vi "Data retrieve engine_SE.vi"(0 "File or Folder Path":path=path "C:/Users/voodoo/Desktop/IV_separat_Vsgsweep_2fields_Vbg-2.8V", 5 "Scan names":string[](array[string]), 7 "IV setup":T2={"# of Vslow"=1, "# Vfast"=1, "#IV Curves at each gate"=2, "B/T offset"=0, "Discard first # curves"=1, "Manual offset"=0}, 9 "index":T3={"A"=3, "B"=4, "C"=2, "D"=4, "E"=3, "N1"=2, "N2"=2, "N3"=3, "N4"=4, "A 1"=8, "A 2"=14, "C 1"=5, "C 2"=1, "E 2"=4}, 11 "Portion of data":cluster{dbl, dbl}(slide)={0.75, 0.25} scale=0.0..1.0, 12 "Decimate point":dbl=1e-10 format="%#_1f", 13 "Extract paramaters from comments?":bool) -> (3 "Comments":string, 4 "IV":cluster{dbl[], dbl[]}[][](array[cluster])=[[{[-2.301174301585294e-09, -2.201174301585294e-09, -2.1011743015852944e-09, -2.0011743015852943e-09, -1.9011743015852942e-09, -1.8011743015852941e-09, -1.701174301585294e-09, -1.601174301585294e-09, -1.5011743015852941e-09, -1.401174301585294e-09, -1.301174301585294e-09, -1.2011743015852942e-09, -1.101174301585294e-09, -1.001174301585294e-09, -9.011743015852942e-10, -8.011743015852941e-10, -7.01174301585294e-10, -6.011743015852942e-10, -5.011743015852941e-10, -4.01174301585294e-10, -3.0117430158529395e-10, -2.0117430158529388e-10, -1.0117430158529423e-10, -1.1743015852941594e-12], [-2.4075285232756958e-05, -1.737972813858452e-05, -1.1037615852397166e-05, -5.267782040080203e-06, 2.4232289247411676e-07, 5.628820057942294e-06, 1.015781505747205e-05, 1.4463328409568988e-05, 1.817222828467457e-05, 2.105509970958606e-05, 2.409775741426245e-05, 2.720796229813868e-05, 3.0197002730537915e-05, 3.3043546244784785e-05, 3.5385544630750595e-05, 3.756777735485851e-05, 3.987253185589809e-05, 4.20620889081888e-05, 4.4006459573108544e-05, 4.587698979226302e-05, 4.7931581768717136e-05, 4.925252522526536e-05, 5.0480327825776546e-05, 8.08077413503745e-08]}]], 6 "IV-2T":cluster{dbl[], dbl[]}[][](array[cluster])=[[{[-2.301174301585294e-09, -2.201174301585294e-09, -2.1011743015852944e-09, -2.0011743015852943e-09, -1.9011743015852942e-09, -1.8011743015852941e-09, -1.701174301585294e-09, -1.601174301585294e-09, -1.5011743015852941e-09, -1.401174301585294e-09, -1.301174301585294e-09, -1.2011743015852942e-09, -1.101174301585294e-09, -1.001174301585294e-09, -9.011743015852942e-10, -8.011743015852941e-10, -7.01174301585294e-10, -6.011743015852942e-10, -5.011743015852941e-10, -4.01174301585294e-10, -3.0117430158529395e-10, -2.0117430158529388e-10, -1.0117430158529423e-10, -1.1743015852941594e-12], [-0.002353462043255516, -0.002297777119659299, -0.002239582947886705, -0.0021846959913649658, -0.0021298090348432263, -0.0020715829478867047, -0.0020166959913649656, -0.0019611544893886803, -0.0019081505368195105, -0.0018609817056506796, -0.0018106102770792509, -0.0017577829478867043, -0.001702609034843226, -0.001644382947886704, -0.001589759034843226, -0.001532834880253854, -0.001467967102476076, -0.0013968026580316317, -0.0013115945420896027, -0.0012138299473531684, -0.00047154515277183454, 0.001680737250983384, 0.0029627659595722446, 4.901687369444213e-06]}]], 8 "Vfast":dbl[][](array[numeric])=[[-1.3]], 10 "Vslow":dbl[](array[numeric])=[-1.3], 14 "N":cluster{"N1":dbl, "N2":dbl, "N3":dbl, "N4":dbl}={"N1"=8999.947, "N2"=0.049942, "N3"=-1.324126602495439e-06, "N4"=0.08912017346699704}, 15 "Vslowest":dbl)   [LabVIEW 2016]
uses:
  <vilib>/addons/WireFlow/_WF_ProgressBar.llb/ProgressBar_WireFlow.lvclass
  <vilib>/Analysis/2dsp.llb/Decimate (single shot, DBL).vi
  <vilib>/Analysis/NI_AALPro.lvlib
panel:
  in  "output array":path[](array[path])
  out "WF-ProgressBar out":refnum<class "ProgressBar_WireFlow.lvclass">
  in  "Tab Control":T1(tab)
  out "IV 2T":cluster{dbl[], dbl[]}[](graph)=[{[-2.301174301585294e-09, -2.201174301585294e-09, -2.1011743015852944e-09, -2.0011743015852943e-09, -1.9011743015852942e-09, -1.8011743015852941e-09, -1.701174301585294e-09, -1.601174301585294e-09, -1.5011743015852941e-09, -1.401174301585294e-09, -1.301174301585294e-09, -1.2011743015852942e-09, -1.101174301585294e-09, -1.001174301585294e-09, -9.011743015852942e-10, -8.011743015852941e-10, -7.01174301585294e-10, -6.011743015852942e-10, -5.011743015852941e-10, -4.01174301585294e-10, -3.0117430158529395e-10, -2.0117430158529388e-10, -1.0117430158529423e-10, -1.1743015852941594e-12], [-0.002353462043255516, -0.002297777119659299, -0.002239582947886705, -0.0021846959913649658, -0.0021298090348432263, -0.0020715829478867047, -0.0020166959913649656, -0.0019611544893886803, -0.0019081505368195105, -0.0018609817056506796, -0.0018106102770792509, -0.0017577829478867043, -0.001702609034843226, -0.001644382947886704, -0.001589759034843226, -0.001532834880253854, -0.001467967102476076, -0.0013968026580316317, -0.0013115945420896027, -0.0012138299473531684, -0.00047154515277183454, 0.001680737250983384, 0.0029627659595722446, 4.901687369444213e-06]}]
  out "IV":cluster{dbl[], dbl[]}[](graph)=[{[-2.301174301585294e-09, -2.201174301585294e-09, -2.1011743015852944e-09, -2.0011743015852943e-09, -1.9011743015852942e-09, -1.8011743015852941e-09, -1.701174301585294e-09, -1.601174301585294e-09, -1.5011743015852941e-09, -1.401174301585294e-09, -1.301174301585294e-09, -1.2011743015852942e-09, -1.101174301585294e-09, -1.001174301585294e-09, -9.011743015852942e-10, -8.011743015852941e-10, -7.01174301585294e-10, -6.011743015852942e-10, -5.011743015852941e-10, -4.01174301585294e-10, -3.0117430158529395e-10, -2.0117430158529388e-10, -1.0117430158529423e-10, -1.1743015852941594e-12], [-2.4075285232756958e-05, -1.737972813858452e-05, -1.1037615852397166e-05, -5.267782040080203e-06, 2.4232289247411676e-07, 5.628820057942294e-06, 1.015781505747205e-05, 1.4463328409568988e-05, 1.817222828467457e-05, 2.105509970958606e-05, 2.409775741426245e-05, 2.720796229813868e-05, 3.0197002730537915e-05, 3.3043546244784785e-05, 3.5385544630750595e-05, 3.756777735485851e-05, 3.987253185589809e-05, 4.20620889081888e-05, 4.4006459573108544e-05, 4.587698979226302e-05, 4.7931581768717136e-05, 4.925252522526536e-05, 5.0480327825776546e-05, 8.08077413503745e-08]}]
  # "Use to extract gate values in comments\neg. Vsg1="
  # "Default:\n4 terminal V vs I \n2 terminal V vs I"
  # "How many curves at each field/temperature? Usually should be N(Vslow)*N(Vfast)*N(each gate)"
  # "Discard first few IV curves at each gate if the gate need\ntime to settle"
  # "Default decimate on current axis instead of voltage axis. Decimation is needed for extracting dV/dI"
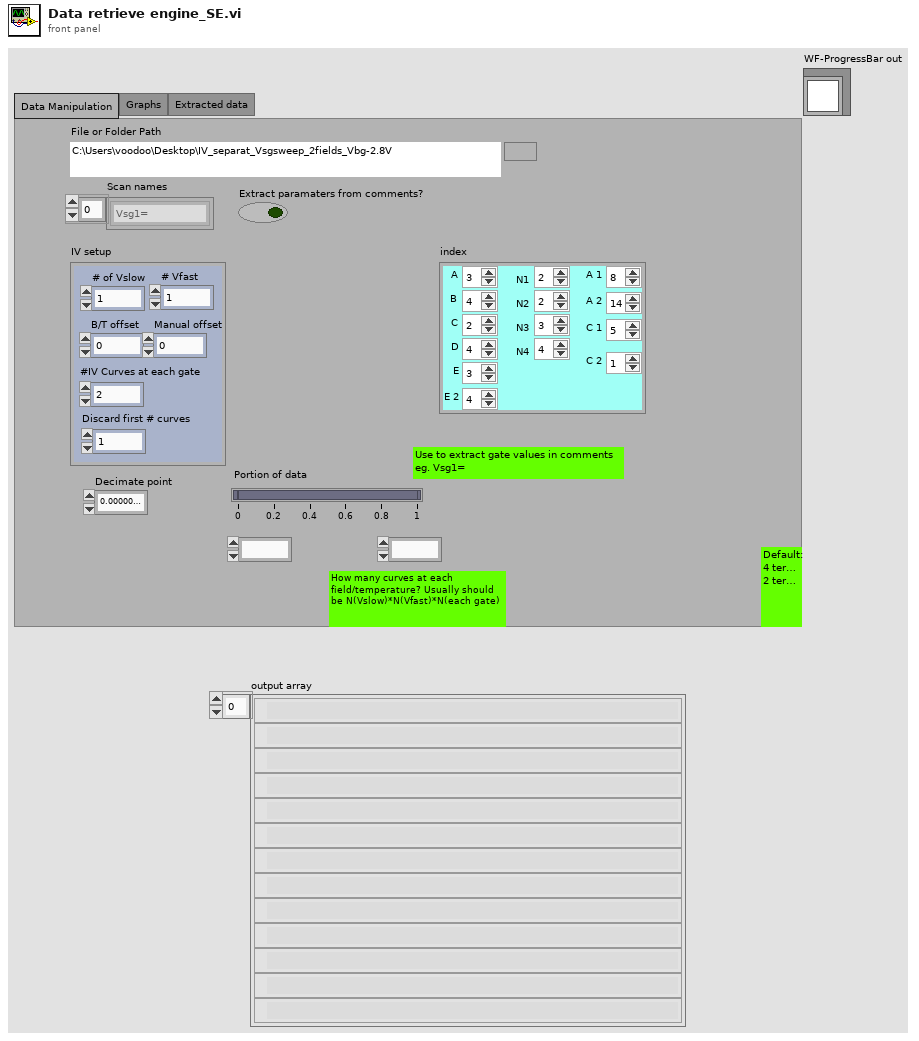
[diagram p1: front panel]
types:
  T1 = enum32{"Data Manipulation", "Graphs", "Extracted data"}
  T2 = cluster{"# of Vslow":i32, "# Vfast":i32, "#IV Curves at each gate":i32, "B/T offset":i32, "Discard first # curves":i32, "Manual offset":i32}
  T3 = cluster{"A":i32, "B":i32, "C":i32, "D":i32, "E":i32, "N1":i32, "N2":i32, "N3":i32, "N4":i32, "A 1":i32, "A 2":i32, "C 1":i32, "C 2":i32, "E 2":i32}
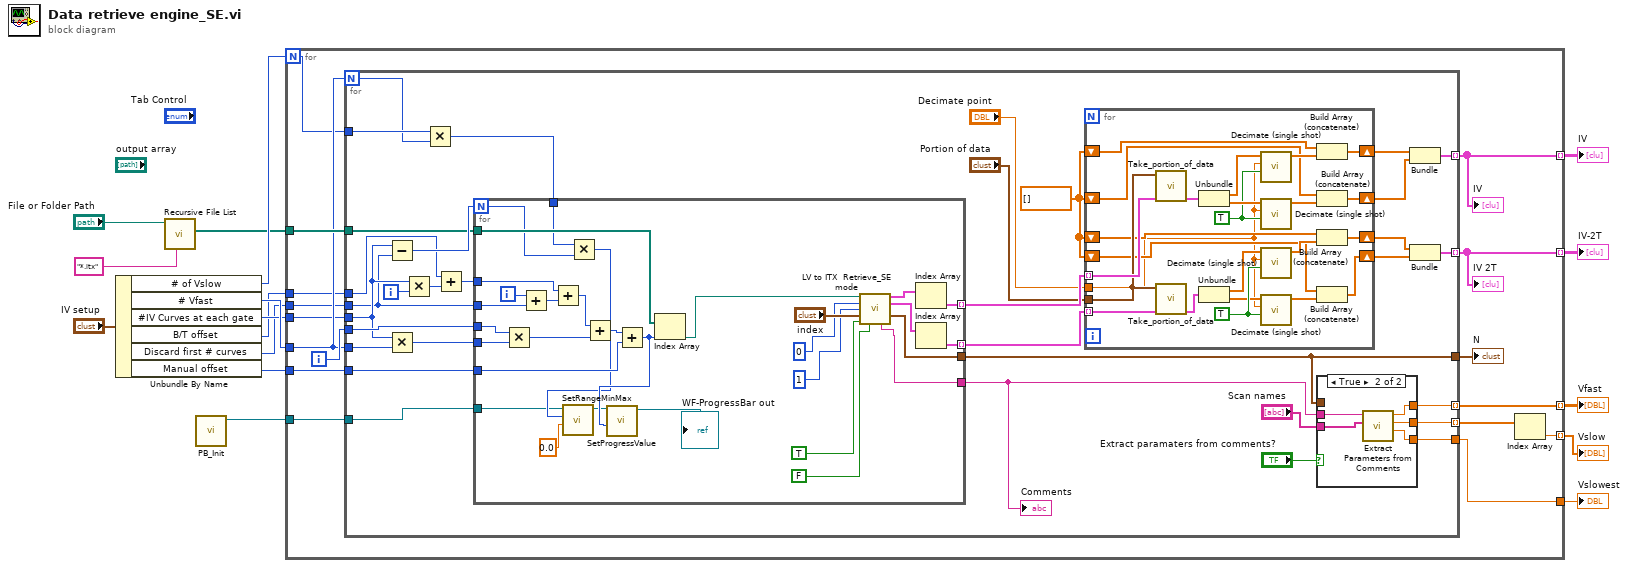
[diagram p0: block diagram]
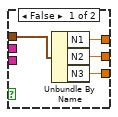
[diagram p2: hidden frame]
diagram:
  n1 = Unbundle By Name("IV setup") -> ("# of Vslow"=w14:i32, "# Vfast"=w13:i32, "#IV Curves at each gate"=w12:i32, "B/T offset"=w10:i32, "Discard first # curves"=w11:i32, "Manual offset"=w9:i32)
  n2 = call <vilib>:"Recursive File List.vi"("pattern"="*.itx", "Folder Path"="File or Folder Path") -> ("All Files in Dir"=w1:path[])  [unwired: 5 in, 4 out]
  n3 = call <vilib>:"PB_Init.vi"() -> ("WF-ProgressBar out"=w2:refnum<class "ProgressBar_WireFlow.lvclass">)  [unwired: 10 in, 1 out]
  n4 = for {
    N: w14 -> [w18]
    tunnel: [w31] -> w16 mode=indexing
    tunnel: w1 -> [w29]
    tunnel: w13 -> [w28]
    tunnel: w12 -> [w27]
    tunnel: w11 -> [w26]
    tunnel: w10 -> [w25]
    tunnel: w9 -> [w24]
    tunnel: [w23] -> w8 mode=indexing
    tunnel: [w22] -> w7 mode=indexing
    tunnel: [w20] -> w6 mode=indexing
    tunnel: [w19] -> w5
    tunnel: w2 -> [w17]
    i -> [w32]
    n5 = for {
      N: w28 -> [w35]
      tunnel: w28 -> [w62]
      tunnel: w32 -> [w61]
      tunnel: [w40] -> w30
      tunnel: w29 -> [w59]
      tunnel: w27 -> [w58]
      tunnel: w26 -> [w57]
      tunnel: w25 -> [w56]
      tunnel: w24 -> [w55]
      tunnel: [w45] -> w22 mode=indexing
      tunnel: [w44] -> w23 mode=indexing
      tunnel: [w37] -> w19
      tunnel: [w43] -> w21 mode=indexing
      tunnel: [w38] -> w20 mode=indexing
      tunnel: w18 -> [w36]
      tunnel: w17 -> [w33]
      i -> [w65]
      w48 = dbl[] []
      n6 = Subtract(x=w58, y=w57) -> (x-y=w60:i32)
      n7 = Multiply(x=w58, y=w62) -> (x*y=w63:i32)
      n8 = Multiply(x=w58, y=w65) -> (x*y=w66:i32)
      n9 = Multiply(x=w36, y=w35) -> (x*y=w34:i32)
      n10 = Add(x=w56, y=w66) -> (x+y=w64:i32)
      n11 = for {
        N: w60 -> [w105]
        tunnel: w64 -> [w130]
        tunnel: [w109] -> w41
        tunnel: w63 -> [w127]
        tunnel: [w126] -> w54 mode=indexing
        tunnel: w61 -> [w124]
        tunnel: [w110] -> w40
        tunnel: w57 -> [w123]
        tunnel: [w122] -> w53 mode=indexing
        tunnel: w59 -> [w121]
        tunnel: w55 -> [w119]
        tunnel: w34 -> [w106]
        tunnel: w33 -> [w103]
        i -> [w108]
        n12 = Multiply(x=w124, y=w127) -> (x*y=w128:i32)
        n13 = Add(x=w108, y=w123) -> (x+y=w125:i32)
        n14 = Add(x=w130, y=w125) -> (x+y=w129:i32)
        n15 = Multiply(x=w106, y=w105) -> (x*y=w104:i32)
        n16 = call-dynamic "SetRangeMinMax.vi"("Min (0)"=0.0, "Max (1)"=w104, "WF-ProgressBar in"=w103) -> ("WF-ProgressBar out"=w101:refnum<class "ProgressBar_WireFlow.lvclass">)  [unwired: 7 in, 1 out]
        n17 = Add(x=w129, y=w128) -> (x+y=w120:i32)
        n18 = Add(x=w120, y=w119) -> (x+y=w107:i32)
        n19 = call-dynamic "SetProgressValue.vi"("Value"=w107, "WF-ProgressBar in"=w101) -> ("WF-ProgressBar out"=→"WF-ProgressBar out":refnum<class "ProgressBar_WireFlow.lvclass">)  [unwired: 7 in, 2 out]
        n20 = Index Array(array=w121, index=w107) -> (element=w115:path)
        n21 = call "LV to ITX  Retrieve_SE mode.vi"("File or Folder Path"=w115, "offset"=0, "length"=1, "index"="index", "stop"=TRUE, "file contains 2D data?"=FALSE ("List folder?")) -> ("A vs B"=w118:cluster{dbl[], dbl[]}[], "C vs D"=w117:cluster{dbl[], dbl[]}[], "N"=w110:cluster{"N1":dbl, "N2":dbl, "N3":dbl, "N4":dbl}, "Comments"=w109:string)  [unwired: 6 out]
        n22 = Index Array(array=w118) -> (element=w126:cluster{dbl[], dbl[]})  [unwired: 1 in]
        n23 = Index Array(array=w117) -> (element=w122:cluster{dbl[], dbl[]})  [unwired: 1 in]
      }
      "Comments" <- w41
      n24 = for {
        tunnel: w54 -> [w99] mode=indexing
        tunnel: w53 -> [w82] mode=indexing
        tunnel: "Portion of data" -> [w81]
        tunnel: "Decimate point" -> [w76]
        shift-right: [w94] -> w50
        shift-left: w48 -> [w92]
        shift-right: [w90] -> w49
        shift-left: w48 -> [w89]
        shift-right: [w80] -> w47
        shift-left: w48 -> [w79]
        shift-right: [w78] -> w46
        shift-left: w48 -> [w77]
        w85 = TRUE ("averaging")
        w96 = TRUE ("averaging")
        n25 = call <userlib>:"Take_portion_of_data.vi"("input IV"=w99, "Slide"=w81) -> ("Output IV"=w95:cluster{dbl[], dbl[]})  [unwired: 5 in]
        n26 = call <userlib>:"Take_portion_of_data.vi"("input IV"=w82, "Slide"=w81) -> ("Output IV"=w86:cluster{dbl[], dbl[]})  [unwired: 5 in]
        n27 = Unbundle(w95) -> (w97:dbl[], w98:dbl[])
        n28 = Unbundle(w86) -> (w84:dbl[], w83:dbl[])
        n29 = call-poly <vilib>:"Decimate (single shot).vi"("averaging"=w96, "decimating factor"=w76, "X"=w97) -> ("Decimated Array"=w93:dbl[])  [unwired: 7 in, 1 out]
        n30 = call-poly <vilib>:"Decimate (single shot).vi"("averaging"=w96, "decimating factor"=w76, "X"=w98) -> ("Decimated Array"=w91:dbl[])  [unwired: 7 in, 1 out]
        n31 = call-poly <vilib>:"Decimate (single shot).vi"("averaging"=w85, "decimating factor"=w76, "X"=w84) -> ("Decimated Array"=w87:dbl[])  [unwired: 7 in, 1 out]
        n32 = call-poly <vilib>:"Decimate (single shot).vi"("averaging"=w85, "decimating factor"=w76, "X"=w83) -> ("Decimated Array"=w88:dbl[])  [unwired: 7 in, 1 out]
        n33 = Build Array (concatenate)(w92, w93) -> (w94:dbl[])
        n34 = Build Array (concatenate)(w89, w91) -> (w90:dbl[])
        n35 = Build Array (concatenate)(w79, w87) -> (w80:dbl[])
        n36 = Build Array (concatenate)(w77, w88) -> (w78:dbl[])
      }
      n37 = case shown="True" "Extract paramaters from comments?" {
        tunnel: [w67 w75] -> w38
        tunnel: [w68 w74] -> w37
        tunnel: [w69 w73] -> w43
        tunnel: "Scan names" -> [_ w72]
        tunnel: w41 -> [_ w71]
        tunnel: w40 -> [w70 _]
        frame False {
          n38 = Unbundle By Name(w70) -> ("N1"=w67:dbl, "N2"=w69:dbl, "N3"=w68:dbl)
        }
        frame True {
          n39 = call <userlib>:"Extract Parameters from Comments.vi"("Scan names"=w72, "Comments"=w71) -> ("Numeric"=w74:dbl, "Numeric 3"=w73:dbl, "Numeric 2"=w75:dbl)  [unwired: 7 in]
        }
      }
      n40 = Bundle(w50, w49) -> (w44:cluster{dbl[], dbl[]})  [unwired: 1 in]
      n41 = Bundle(w47, w46) -> (w45:cluster{dbl[], dbl[]})  [unwired: 1 in]
    }
    "IV" <- w23
    "N" <- w30
    "IV 2T" <- w22
    n42 = Index Array(array=w21) -> (element=w31:dbl)  [unwired: 1 in]
  }
  "Vslow" <- w16
  "Vfast" <- w6
  "IV" <- w8
  "IV-2T" <- w7
  "Vslowest" <- w5
